vi "unused_Read controlTerminals.vi"(8 "error in (no error)":errorcluster, 11 "BlockDiagram in":refnum<class "BlockDiagram.lvclass">) -> (0 "error out":errorcluster, 2 "terminals":refnum<class "Terminal.lvclass">[](array[class]), 3 "BlockDiagram out":refnum<class "BlockDiagram.lvclass">)   [LabVIEW 2023]
uses:
  BlockDiagram.lvclass/BlockDiagram.ctl
  ControlTerminal/ControlTerminal.lvclass
  C:/projects/TLC_Scripto/Source/Terminal/Terminal.lvclass
  C:/projects/TLC_Scripto/Source/GObject/GObject.lvclass
  C:/projects/TLC_Scripto/Source/Generic/Generic.lvclass
  C:/projects/TLC_Scripto/Source/ControlTerminal/ControlTerminal.lvclass
  BlockDiagram.lvclass
  Terminal/Terminal.lvclass
panel:
  out "Array":string[](array[string])
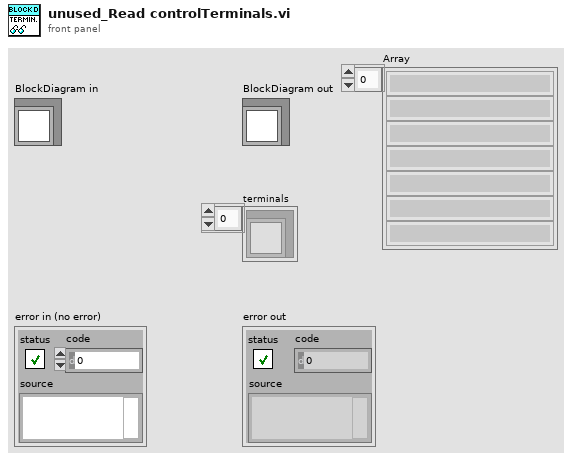
[diagram p1: front panel]
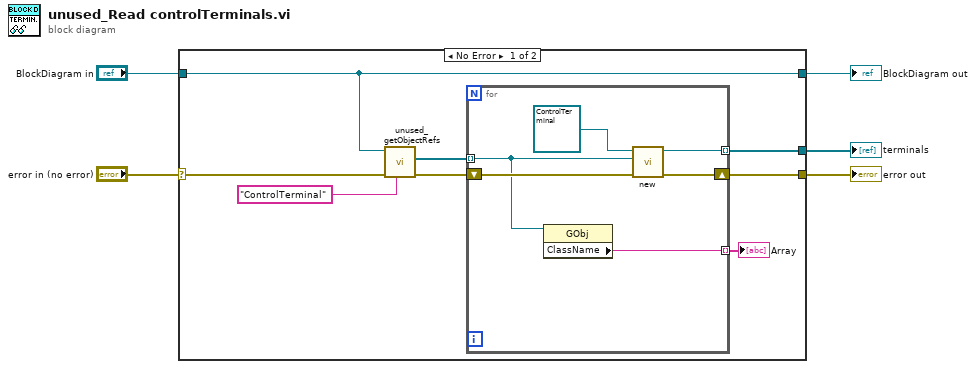
[diagram p0: block diagram]
diagram:
  n1 = case shown="No Error" "error in (no error)" {
    selector: "error in (no error)" -> [w8 w21]
    tunnel: [w10 w21] -> w4
    tunnel: [w11 w20] -> w2
    tunnel: "BlockDiagram in" -> [w11 w20]
    tunnel: [w9 _] -> w1
    frame No Error {
      n2 = call "unused_getObjectRefs.vi"("type(ClassName)"="ControlTerminal", "error in (no error)"=w8, "BlockDiagram in"=w11) -> ("error out"=w12:errorcluster, "refs"=w13:refnum<vi>[])  [unwired: 6 in, 1 out]
      n3 = for {
        tunnel: w13 -> [w15] mode=indexing
        shift-right: [w18] -> w10
        shift-left: w12 -> [w19]
        tunnel: [w17] -> w9 mode=indexing
        tunnel: [w14] -> w6 mode=indexing
        n4 = property class="GObj"(reference=w15) -> ("ClassName"=w14:string)  [unwired: 1 in, 2 out]
        n5 = call-dynamic "new.vi"("Error In"=w19, "ref"=w15, "Generic In"=refnum<class "ControlTerminal.lvclass"> refnum ("TLC_Scripto.lvlib:ControlTerminal")) -> ("Error Out"=w18:errorcluster, "Generic Out"=w17:refnum<class "ControlTerminal.lvclass">)  [unwired: 7 in]
      }
      "Array" <- w6
    }
    frame Error {
    }
  }
  "error out" <- w4
  "BlockDiagram out" <- w2
  "terminals" <- w1
